vi "Log Assert Core.vi"(0 "Assert Name":string, 1 "Data Value":variant, 2 "Status":bool, 3 "Assert VI Name":string, 4 "Calling VI Name":string, 5 "Top Level VI Name":string, 6 "Failure Action":string, 7 "Assert Builder User Name":string, 8 "Last Update":timestamp, 9 "Assert Build Timestamp":timestamp, 10 "Evaluation String":string, 11 "Assert VI UID":i32, 12 "Comment":string, 13 "VI References":T1, 14 "Data Type":string) -> ()   [LabVIEW 2016, in "Assert API Components.lvlib"]
doc: "Core VI which logs all information for each assert and is scripted into each new assert vi.\nSet to Shared Clone Reentrant execution to prevent the assert API causing threadblocks within large applications."
uses:
  Assert API Components.lvlib
  VI References.ctl
  Message Data.ctl
  Log Assert Core Components/Log Assert Core.lvlib
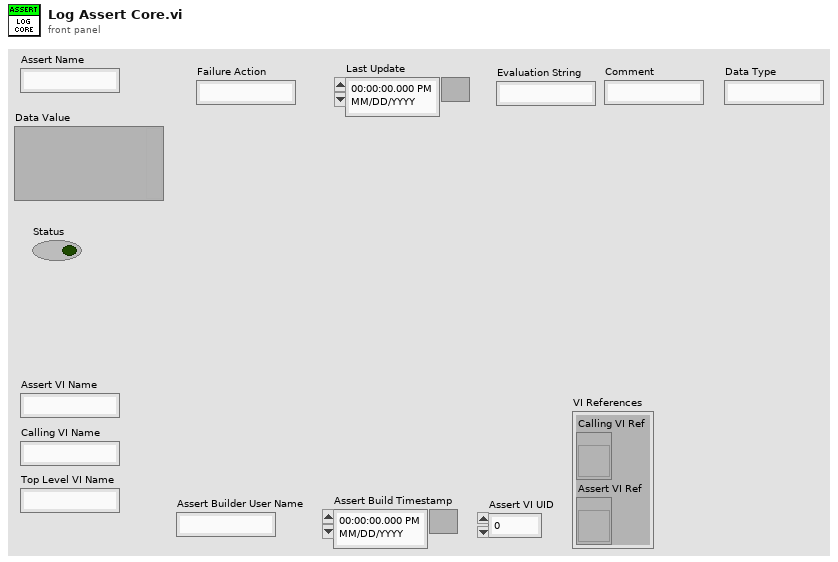
[diagram p1: front panel]
types:
  T1 = typedef "Assert API Components.lvlib/VI References.ctl" = cluster{"Calling VI Ref":refnum<vi>, "Assert VI Ref":refnum<vi>}
  T2 = typedef "Assert API Components.lvlib/Message Data.ctl" = cluster{"Data Value":variant, "Last Update":timestamp, "Comment":string, "Evaluation String":string, "Status":bool, "Assert Name":string, "Failure Action":string, "Assert VI Name":string, "Calling VI Name":string, "Assert VI UID":i32, "Top Level VI Name":string, "VI References":T1, "Assert Build Timestamp":timestamp, "Assert Builder User Name":string, "Data Type":string}
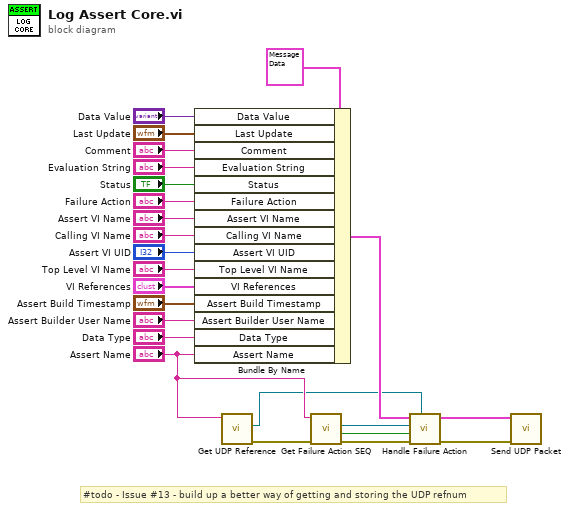
[diagram p0: block diagram]
diagram:
  # "#todo - Issue #13 - build up a better way of getting and storing the UDP refnum"
  n1 = Bundle By Name(cluster=T2 {"Data Value"=variant, "Last Update"=timestamp(0 s since 1904-01-01), "Comment"="", "Evaluation String"="", "Status"=FALSE, "Assert Name"="", "Failure Action"="", "Assert VI Name"="", "Calling VI Name"="", "Assert VI UID"=0, "Top Level VI Name"="", "VI References"={"Calling VI Ref"=refnum, "Assert VI Ref"=refnum}, "Assert Build Timestamp"=timestamp(0 s since 1904-01-01), "Assert Builder User Name"="", "Data Type"=""} ("Assert Message"), "Data Value"="Data Value", "Last Update"="Last Update", "Comment"="Comment", "Evaluation String"="Evaluation String", "Status"="Status", "Failure Action"="Failure Action", "Assert VI Name"="Assert VI Name", "Calling VI Name"="Calling VI Name", "Assert VI UID"="Assert VI UID", "Top Level VI Name"="Top Level VI Name", "VI References"="VI References", "Assert Build Timestamp"="Assert Build Timestamp", "Assert Builder User Name"="Assert Builder User Name", "Data Type"="Data Type", "Assert Name"="Assert Name") -> (w4:T2)
  n2 = call "Get UDP Reference.vi"("Assert Name"="Assert Name") -> ("error out"=w9:errorcluster, "UDP Reference"=w3:refnum<k16>)  [unwired: 9 in]
  n3 = call "Get Failure Action SEQ.vi"("error in (no error)"=w9, "Assert Name"="Assert Name") -> ("error out"=w8:errorcluster, "created new?"=w7:bool, "Assert FA SEQ"=w6:refnum<queue>)  [unwired: 7 in]
  n4 = call "Handle Failure Action.vi"("UDP Port"=w3, "error in (no error)"=w8, "Created New"=w7, "Assert FA SEQ"=w6, "Assert Message in"=w4) -> ("error out"=w2:errorcluster, "Assert Message out"=w1:T2)  [unwired: 5 in]
  n5 = call "Send UDP Packet.vi"("error in (no error)"=w2, "Assert Message in"=w1) -> ()  [unwired: 9 in, 1 out]
